vi "test_CalculateSpecificationBuildOrder_DynamicDispatchAssetsSolution.vi"() -> (3 "Pass?":bool)   [LabVIEW 2019, in "Tests.SolutionBuilder.lvlib"]
uses:
  Tests.SolutionBuilder.lvlib
  SolutionBuilder/SolutionBuilder.lvclass
  SolutionBuilder/ProjectItem/ProjectItem.lvclass
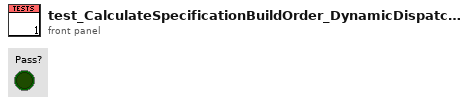
[diagram p1: front panel]
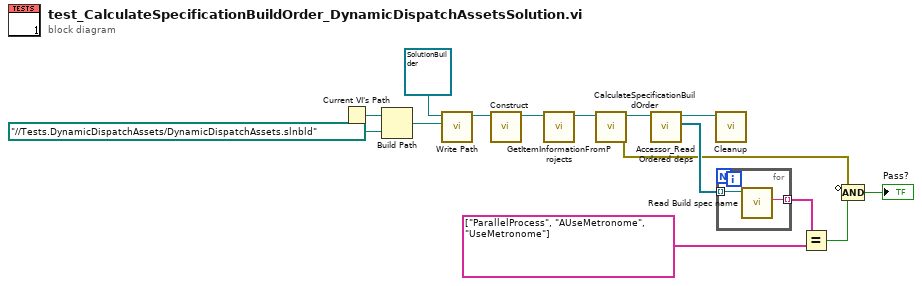
[diagram p0: block diagram]
diagram:
  n1 = Current VI's Path() -> (path=w15:path)
  n2 = Build Path(base path=w15, name or relative path=path "../../Tests.DynamicDispatchAssets/DynamicDispatchAssets.slnbld" ("Path")) -> (appended path=w13:path)
  n3 = call "Write Path.vi"("Path"=w13, "SolutionBuilder in"=refnum<class "SolutionBuilder.lvclass"> refnum) -> ("SolutionBuilder out"=w12:refnum<class "SolutionBuilder.lvclass">)  [unwired: 9 in]
  n4 = call "Construct.vi"("SolutionBuilder in"=w12) -> ("SolutionBuilder out"=w10:refnum<class "SolutionBuilder.lvclass">)  [unwired: 9 in, 1 out]
  n5 = call "GetItemInformationFromProjects.vi"("SolutionBuilder in"=w10) -> ("SolutionBuilder out"=w9:refnum<class "SolutionBuilder.lvclass">)  [unwired: 9 in, 1 out]
  n6 = call "CalculateSpecificationBuildOrder.vi"("SolutionBuilder in"=w9) -> ("error out"=w5:errorcluster, "SolutionBuilder out"=w8:refnum<class "SolutionBuilder.lvclass">)  [unwired: 9 in]
  n7 = call "Accessor_Read Ordered deps.vi"("SolutionBuilder in"=w8) -> ("Ordered deps"=w6:refnum<class "ProjectItem.lvclass">[], "SolutionBuilder out"=w7:refnum<class "SolutionBuilder.lvclass">)  [unwired: 8 in, 1 out]
  n8 = call "Cleanup.vi"("SolutionBuilder in"=w7) -> ()  [unwired: 9 in, 2 out]
  n9 = for {
    tunnel: w6 -> [w17] mode=indexing
    tunnel: [w16] -> w4 mode=indexing
    n10 = call "Read Build spec name.vi"("ProjectItem in"=w17) -> ("Build spec name"=w16:string)  [unwired: 9 in, 1 out]
  }
  n11 = Equal?(x=w4, y=string[] ["ParallelProcess", "AUseMetronome", "UseMetronome"] ("Array")) -> (x = y?=w11:bool)
  n12 = Compound Arithmetic op=AND(invert w5, w11) -> (→"Pass?":bool)
